vi "On Compile - Group Hardware Channels by Message Type.vi"(8 "error in":errorcluster, 11 "hardware channel data":T3[](array[typedef]) {"labels settings for RT"."Label Timestamp Channel Data Reference" format="%.0x"; "labels settings for RT"."Word Initial Raw Value" format="%032.0f"; "labels settings for RT"."Label Disable/Trigger Channel Reference" format="%.0x"; "labels settings for RT"."parameter driver data"."Tx parameter refs" format="%.0x"; "labels settings for RT"."parameter driver data"."Rx block data refs"."Data Reference" format="%.0x"; "labels settings for RT"."SDI" format="%02b"; "labels settings for RT"."label" format="%.0o"}) -> (0 "error out":errorcluster, 3 "grouped hardware channel data refs":T2(array[cluster]) {"VS Refs" format="%.0x"})   [LabVIEW 2020, in "Ballard ARINC 429 System Explorer.lvlib" / "Implementation.lvlib"]
uses:
  Implementation.lvlib
  Shared/RT Hardware Channel Settings.ctl
  Shared/RT Label Settings.ctl
  Shared/Label.ctl
  Shared/RT Parameters.ctl
  Shared/Parameter Definition.ctl
  Encoding and Decoding/Encoding.ctl
  <vilib>/NI VeriStand/Custom Device API/Block Data Reference.ctl
  <vilib>/NI VeriStand/Custom Device API/Data Reference.ctl
  <vilib>/NI VeriStand/Custom Device API/Custom Device Item Ref.ctl
  Shared/Transfer Type.ctl
  <vilib>/NI VeriStand/Custom Device API/Custom Device API.lvlib
  Encoding and Decoding/Encoding and Decoding.lvlib
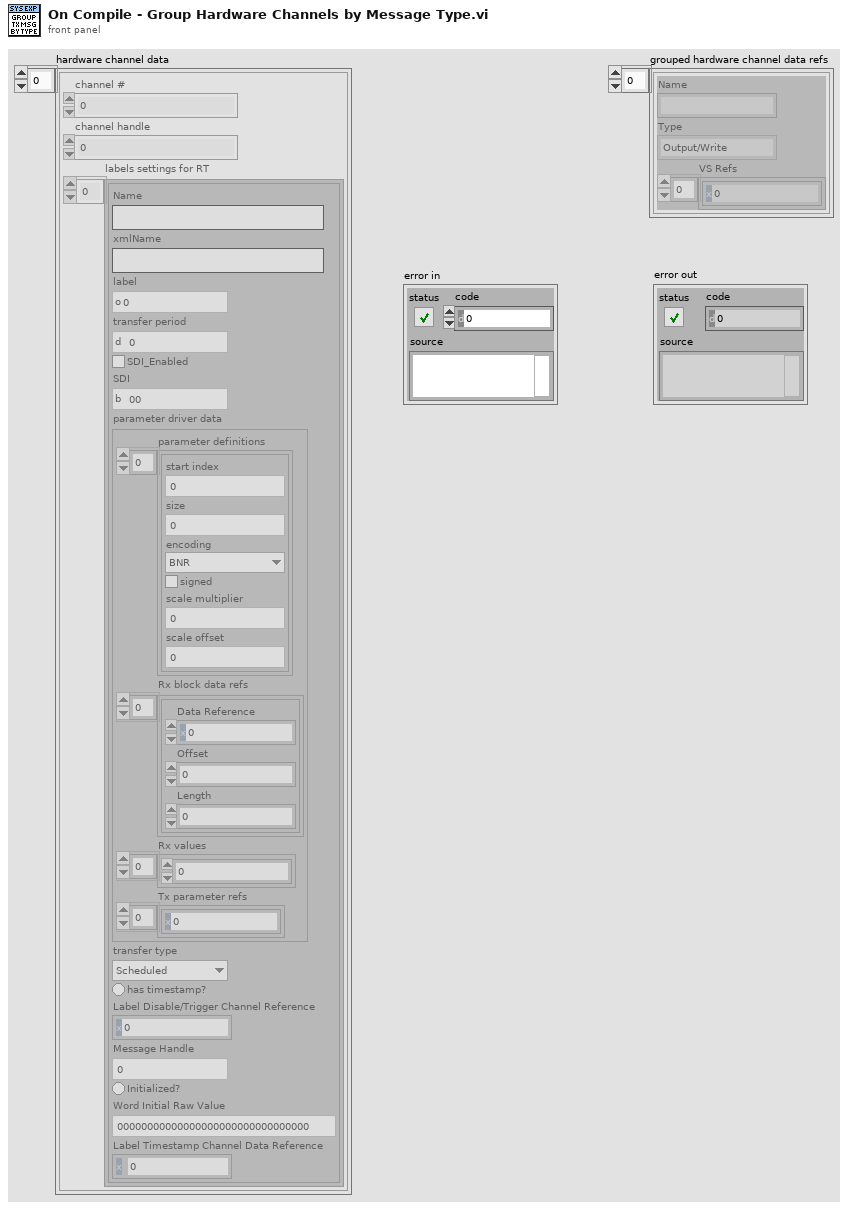
[diagram p1: front panel]
types:
  T1 = typedef "Custom Device API.lvlib/Custom Device Item Ref.ctl" = u64
  T2 = cluster{"Name":string, "Type":enum16{"Output/Write", "Input/Read", "Input/ReadWrite"}, "VS Refs":T1[]}[]
  T3 = typedef "RT Hardware Channel Settings.ctl" = cluster{"channel #":u16, "channel handle":u64, "labels settings for RT":T4[]}
  T4 = typedef "RT Label Settings.ctl" = cluster{"Name":string, "xmlName":string, "label":T5, "transfer period":u32, "SDI_Enabled":bool, "SDI":u8, "parameter driver data":T6, "transfer type":T11, "has timestamp?":bool, "Label Disable/Trigger Channel Reference":T1, "Message Handle":u64, "Initialized?":bool, "Word Initial Raw Value":u32, "Label Timestamp Channel Data Reference":T10}
  T5 = typedef "Label.ctl" = u8
  T6 = typedef "RT Parameters.ctl" = cluster{"parameter definitions":T7[], "Rx block data refs":T9[], "Rx values":dbl[], "Tx parameter refs":T1[]}
  T7 = typedef "Parameter Definition.ctl" = cluster{"start index":i32, "size":i32, "encoding":T8, "signed":bool, "scale multiplier":dbl, "scale offset":dbl}
  T8 = typedef "Encoding and Decoding.lvlib/Encoding.ctl" = enum16{"BNR", "BCD", "Discrete"}
  T9 = typedef "Custom Device API.lvlib/Block Data Reference.ctl" = cluster{"Data Reference":T10, "Offset":u64, "Length":u64}
  T10 = typedef "Custom Device API.lvlib/Data Reference.ctl" = i32
  T11 = typedef "Transfer Type.ctl" = enum16{"Scheduled", "Acyclic", "Block", "Strobe"}
  T12 = cluster{"Group":cluster{"Name":string, "Type":enum16{"Output/Write", "Input/Read", "Input/ReadWrite"}, "VS Refs":T1[]}, "transfer type":T11}[]
  T13 = cluster{"Name":string, "Type":enum16{"Output/Write", "Input/Read", "Input/ReadWrite"}, "VS Refs":T1[]}
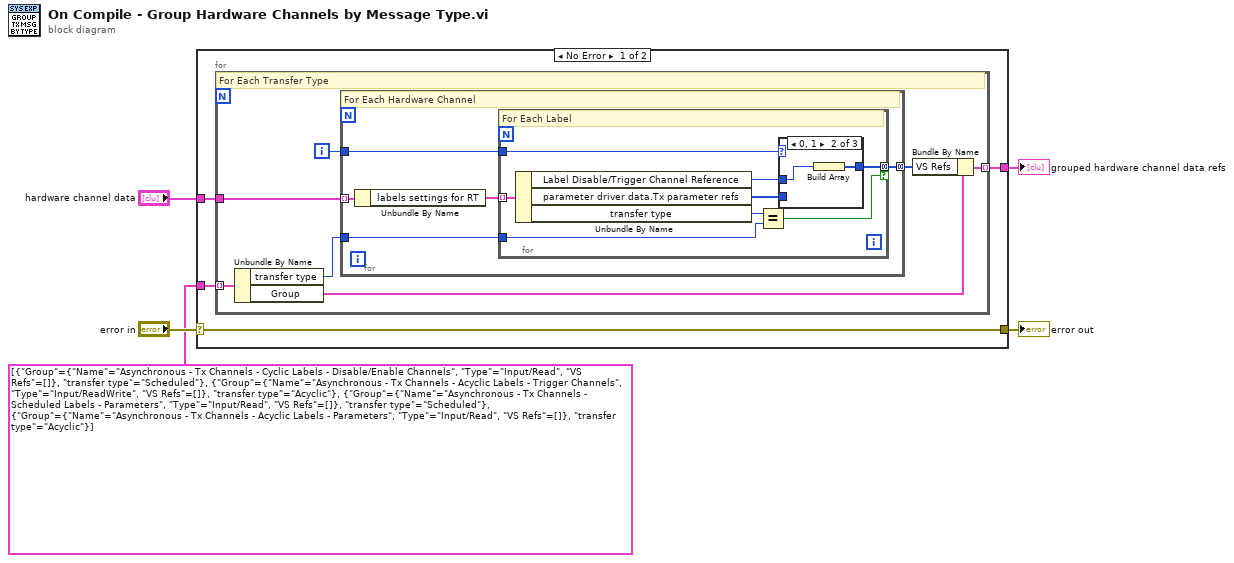
[diagram p0: block diagram]
diagram:
  n1 = case shown="No Error" "error in" {
    selector: "error in" -> [w8 w33]
    tunnel: "hardware channel data" -> [w9 _]
    tunnel: [w8 w33] -> w3
    tunnel: T12 [{"Group"={"Name"="Asynchronous - Tx Channels - Cyclic Labels - Disable/Enable Channels", "Type"=enum."Input/Read", "VS Refs"=[]}, "transfer type"=enum."Scheduled"}, {"Group"={"Name"="Asynchronous - Tx Channels - Acyclic Labels - Trigger Channels", "Type"=enum."Input/ReadWrite", "VS Refs"=[]}, "transfer type"=enum."Acyclic"}, {"Group"={"Name"="Asynchronous - Tx Channels - Scheduled Labels - Parameters", "Type"=enum."Input/Read", "VS Refs"=[]}, "transfer type"=enum."Scheduled"}, {"Group"={"Name"="Asynchronous - Tx Channels - Acyclic Labels - Parameters", "Type"=enum."Input/Read", "VS Refs"=[]}, "transfer type"=enum."Acyclic"}] -> [w7 _]
    tunnel: [w6 _] -> w1
    frame No Error {
      n2 = for {
        tunnel: w9 -> [w16]
        tunnel: w7 -> [w15] mode=indexing
        tunnel: [w10] -> w6 mode=indexing
        i -> [w13]
        # "For Each Transfer Type"
        n3 = Unbundle By Name(w15) -> ("transfer type"=w14:T11, "Group"=w12:T13)
        n4 = for {
          tunnel: w16 -> [w21] mode=indexing
          tunnel: w14 -> [w19]
          tunnel: w13 -> [w18]
          tunnel: [w17] -> w11 mode=concatenating
          # "For Each Hardware Channel"
          n5 = Unbundle By Name(w21) -> ("labels settings for RT"=w20:T4[])
          n6 = for {
            tunnel: w20 -> [w29] mode=indexing
            tunnel: w19 -> [w27]
            tunnel: w18 -> [w26]
            tunnel: [w25] -> w17 mode=concatenating if=w24
            # "For Each Label"
            n7 = Unbundle By Name(w29) -> ("Label Disable/Trigger Channel Reference"=w23:T1, "parameter driver data.Tx parameter refs"=w22:T1[], "transfer type"=w28:T11)
            n8 = Equal?(x=w28, y=w27) -> (x = y?=w24:bool)
            n9 = case shown="0, 1" w26 {
              tunnel: [_ w31 w32] -> w25
              tunnel: w23 -> [_ w30 _]
              tunnel: w22 -> [_ _ w32]
              frame Default {
              }
              frame 0, 1 {
                n10 = Build Array(w30) -> (w31:T1[])
              }
              frame 2, 3 {
              }
            }
          }
        }
        n11 = Bundle By Name(cluster=w12, "VS Refs"=w11) -> (w10:T13)
      }
    }
    frame Error {
    }
  }
  "error out" <- w3
  "grouped hardware channel data refs" <- w1
